vi "Post Build Icon Editor (BuildNIPackage).vi"(5 "Files Generated by Build":path[](array[path]), 6 "Top Level/Always Included VIs":path[](array[path]), 7 "Destination Path":path, 8 "error in (no error)":errorcluster, 9 "Target Name":string, 10 "Build Specification Name":string, 11 "Project Path":path) -> (0 "error out":errorcluster)   [LabVIEW 2021]
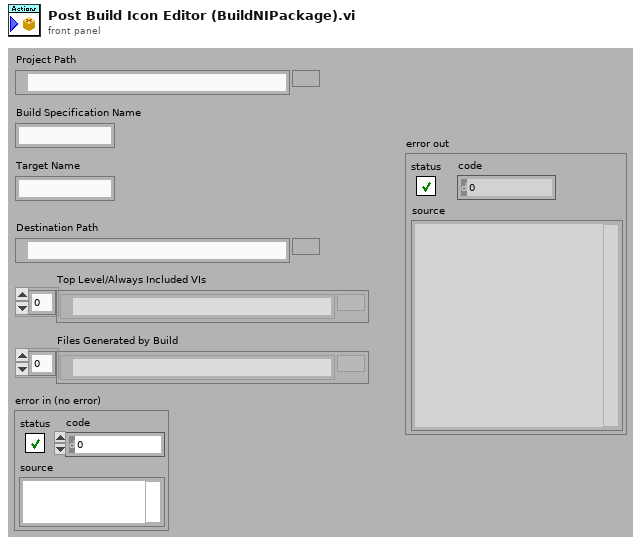
[diagram p1: front panel]
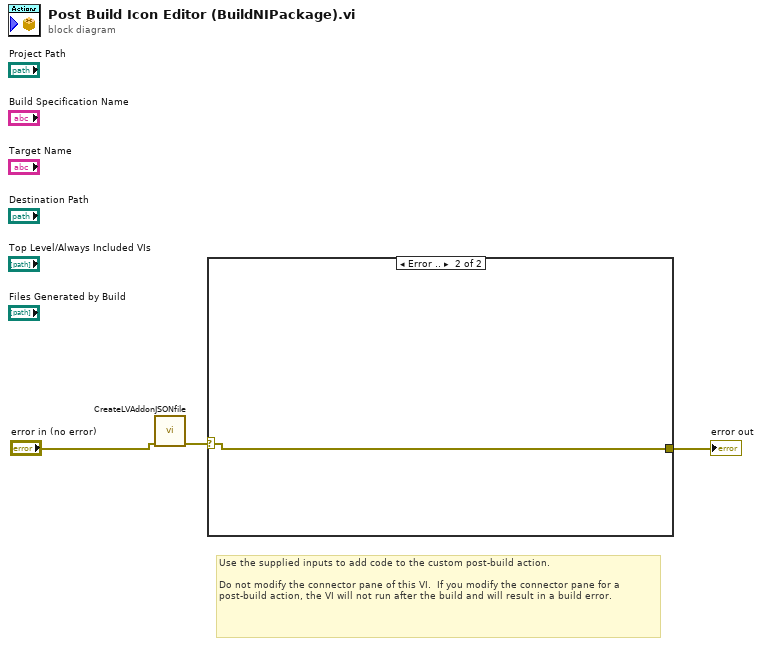
[diagram p0: block diagram]
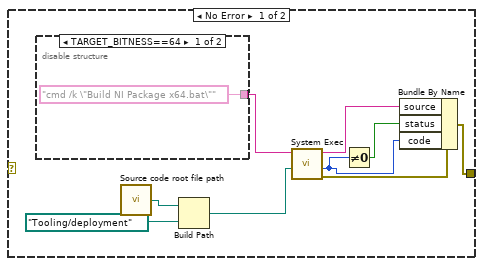
[diagram p2: hidden frame]
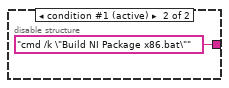
[diagram p3: hidden frame]
diagram:
  # "Use the supplied inputs to add code to the custom post-build action.\n\nDo not modify the connector pane of this VI.  If you modify the connector pane for a post-build action, the VI will not run after the build and will result in a build error."
  n1 = call "CreateLVAddonJSONfile.vi"("error in"="error in (no error)") -> ("error out"=w1:errorcluster)  [unwired: 8 in, 2 out]
  n2 = case shown="Error .." w1 {
    selector: w1 -> [_ w15]
    tunnel: [w5 w15] -> w3
    frame No Error {
      n3 = disable-structure shown="TARGET_BITNESS==64" {
        disable-tunnel: ["cmd /k \"Build NI Package x64.bat\"" ("command line") "cmd /k \"Build NI Package x86.bat\"" ("command line")] -> w12
        frame condition #0 {
        }
        frame condition #1 (active) {
        }
      }
      n4 = call "Source code root file path.vi"() -> ("Source code root path"=w11:path)  [unwired: 1 in]
      n5 = Build Path(base path=w11, name or relative path=path "Tooling/deployment" ("working directory")) -> (appended path=w9:path)
      n6 = call <vilib>:"System Exec.vi"("working directory"=w9, "command line"=w12) -> ("error out"=w8:errorcluster, "return code"=w4:i32, "standard output"=w6:string)  [unwired: 6 in, 1 out]
      n7 = Not Equal To 0?(x=w4) -> (x != 0?=w7:bool)
      n8 = Bundle By Name(cluster=w8, "source"=w6, "status"=w7, "code"=w4) -> (w5:errorcluster)
    }
    frame Error {
    }
  }
  "error out" <- w3
